vi "Last Ack Created Queue.vi"(10 "Queue":refnum<class "Queue.lvclass">, 11 "Base Queue in":refnum<class "Base Queue.lvclass">) -> (3 "Base Queue out":refnum<class "Base Queue.lvclass">)   [LabVIEW 2021, in "jettl.lvlib" / "Base Queue.lvlib" / "Base Queue.lvclass"]
uses:
  Base Queue.lvclass
  Queue/Queue.lvclass
  Base Queue.lvclass/Base Queue.ctl
  Addresses/Addresses.lvlib
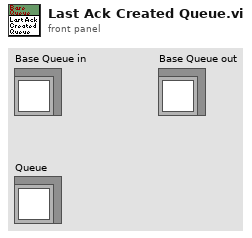
[diagram p1: front panel]
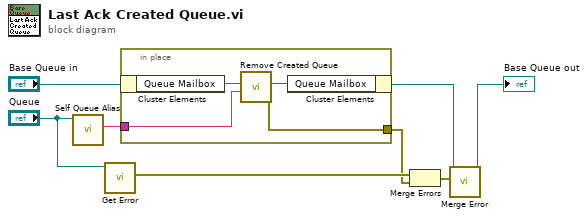
[diagram p0: block diagram]
diagram:
  n1 = call-dynamic "Self Queue Alias.vi"("Queue in"="Queue") -> ("Self Queue Alias"=w1:string)  [unwired: 10 in]
  n2 = call-dynamic "Get Error.vi"("jettl in"="Queue") -> ("Error"=w8:errorcluster)  [unwired: 10 in]
  n3 = in-place {
    in-place-border: w1 -> [w10]
    in-place-border: [w9] -> w3
    n4 = in-place-cluster #1("Base Queue in") -> ("Queue Mailbox"=w12:refnum<data-value>)
    n5 = call "Remove Created Queue.vi"("Self Queue Alias"=w10, "Queue Mailbox in"=w12) -> ("error out"=w9:errorcluster, "Queue Mailbox out"=w11:refnum<data-value>)  [unwired: 8 in]
    n6 = in-place-cluster #1("Queue Mailbox"=w11) -> (w7:refnum<class "Base Queue.lvclass">)
  }
  n7 = Merge Errors(w8, w3) -> (w4:errorcluster)
  n8 = call-dynamic "Merge Error.vi"("Error"=w4, "Base Queue in"=w7) -> ("Base Queue out"=→"Base Queue out":refnum<class "Base Queue.lvclass">)  [unwired: 9 in]
